vi "subReplaceSourceLibaryWithBuiltLibCore.vi"(8 "error in (no error)":errorcluster, 9 "path in":path, 10 "GetProjectItemRefForFile":refnum<vi>, 11 "TargetItem in":refnum<vi>) -> (0 "error out":errorcluster, 1 "Modified Libraries":refnum<vi>[](array[refnum]), 2 "Modified VIs":refnum<vi>[](array[refnum]), 3 "TargetItem out":refnum<vi>)   [LabVIEW 2019, in "SolutionBuilder.lvlib" / "BuildManager.lvclass"]
uses:
  BuildManager.lvclass
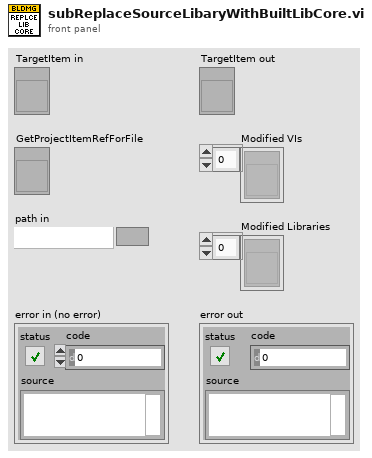
[diagram p1: front panel]
types:
  T1 = enum32{"Save All Without Prompts", "Save All With Prompts", "Do Not Save (Retain In Memory)"}
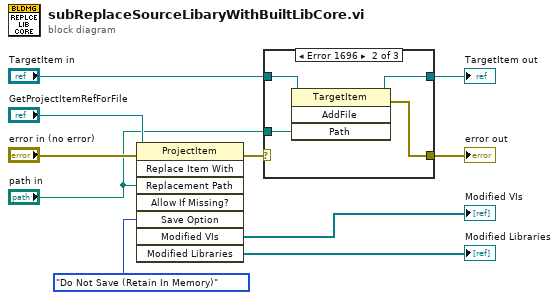
[diagram p0: block diagram]
diagram:
  n1 = invoke class="ProjectItem" method="Replace Item With"(reference="GetProjectItemRefForFile", error in="error in (no error)", "Replacement Path"="path in", "Save Option"=T1."Do Not Save (Retain In Memory)") -> (error out=w5:errorcluster, "Modified VIs"=→"Modified VIs":refnum<vi>[], "Modified Libraries"=→"Modified Libraries":refnum<vi>[])  [unwired: 4 in, 5 out]
  n2 = case shown="Error 1696" w5 {
    selector: w5 -> [w11 _ w17]
    tunnel: "TargetItem in" -> [w12 w16 w18]
    tunnel: "path in" -> [_ w15 _]
    tunnel: [w12 w14 w18] -> w2
    tunnel: [w11 w13 w17] -> w1
    frame No Error {
    }
    frame Error {
      n3 = invoke class="TargetItem" method="AddFile"(reference=w16, "Path"=w15) -> (reference out=w14:refnum<vi>, error out=w13:errorcluster)  [unwired: 2 in, 2 out]
    }
    frame Default {
    }
  }
  "TargetItem out" <- w2
  "error out" <- w1
